vi "MecaDrivePoseEst2_Update.vi"(6 "Time":dbl=-1.0 format="%33.4f", 9 "module Positions":T1 {"RearRight" format="%19.3f"; "RearLeft" format="%19.3f"; "FrontRight" format="%19.3f"; "FrontLeft" format="%19.3f"}, 10 "GyroAngle":T4={"VALUE"=0.0, "COS"=1.0, "SIN"=0.0} {"SIN" format="%13.4f"; "COS" format="%13.4f"; "VALUE" format="%13.4f"}, 11 "in MecaDrivePoseEstimate":T5={"M_Vision_K"=[], "m_nominal_dT"=0.0, "m_PrevTime_Sec"=0.0, "Pose_Buffer"={"TimeStamps"=[], "DataArray"=[], "Min_TimeStamp"=0.0, "Max_TimeStamp"=0.0, "ItemCount"=0, "MaxBufferTime"=0.0}, "Meca_Drive_Odom"={"POSE"={"TRANSLATION"={"X"=0.0, "Y"=0.0}, "ROTATION"={"VALUE"=0.0, "COS"=1.0, "SIN"=0.0}}, "GyroOffset"={"VALUE"=0.0, "COS"=1.0, "SIN"=0.0}, "PreviousAngle"={"VALUE"=0.0, "COS"=1.0, "SIN"=0.0}, "Kinematics"={"FrontLeft"={"X"=0.0, "Y"=0.0}, "FrontRight"={"X"=0.0, "Y"=0.0}, "RearLeft"={"X"=0.0, "Y"=0.0}, "RearRight"={"X"=0.0, "Y"=0.0}, "InverseKinematics"=[[0.0, 1.0, -1.0, 0.0], [0.0, 1.0, 1.0, 0.0], [0.0, 1.0, 1.0, 0.0], [0.0, 1.0, -1.0, 0.0]], "ForwardKinematics"=[[0.0, 1.0, -1.0, 0.0], [0.0, 1.0, 1.0, 0.0], [0.0, 1.0, 1.0, 0.0], [0.0, 1.0, -1.0, 0.0]], "PrevCoR"={"X"=0.0, "Y"=0.0}}, "PreviousWheelPositions"={"FrontLeft"=0.0, "FrontRight"=0.0, "RearLeft"=0.0, "RearRight"=0.0, "P"=FALSE}}, "M_Q"=[[0.0], [0.0], [0.0]]} {"Meca_Drive_Odom"."PreviousWheelPositions"."RearRight" format="%19.3f"; "Meca_Drive_Odom"."PreviousWheelPositions"."RearLeft" format="%19.3f"; "Meca_Drive_Odom"."PreviousWheelPositions"."FrontRight" format="%19.3f"; "Meca_Drive_Odom"."PreviousWheelPositions"."FrontLeft" format="%19.3f"; "Meca_Drive_Odom"."Kinematics"."PrevCoR"."Y" format="%14.3f"; "Meca_Drive_Odom"."Kinematics"."PrevCoR"."X" format="%14.3f"; "Meca_Drive_Odom"."Kinematics"."RearRight"."Y" format="%14.3f"; "Meca_Drive_Odom"."Kinematics"."RearRight"."X" format="%14.3f"; "Meca_Drive_Odom"."Kinematics"."RearLeft"."Y" format="%14.3f"; "Meca_Drive_Odom"."Kinematics"."RearLeft"."X" format="%14.3f"; "Meca_Drive_Odom"."Kinematics"."FrontRight"."Y" format="%14.3f"; "Meca_Drive_Odom"."Kinematics"."FrontRight"."X" format="%14.3f"; "Meca_Drive_Odom"."Kinematics"."FrontLeft"."Y" format="%14.3f"; "Meca_Drive_Odom"."Kinematics"."FrontLeft"."X" format="%14.3f"; "Meca_Drive_Odom"."PreviousAngle"."SIN" format="%13.4f"; "Meca_Drive_Odom"."PreviousAngle"."COS" format="%13.4f"; "Meca_Drive_Odom"."PreviousAngle"."VALUE" format="%13.4f"; "Meca_Drive_Odom"."GyroOffset"."SIN" format="%13.4f"; "Meca_Drive_Odom"."GyroOffset"."COS" format="%13.4f"; "Meca_Drive_Odom"."GyroOffset"."VALUE" format="%13.4f"; "Meca_Drive_Odom"."POSE"."ROTATION"."SIN" format="%13.4f"; "Meca_Drive_Odom"."POSE"."ROTATION"."COS" format="%13.4f"; "Meca_Drive_Odom"."POSE"."ROTATION"."VALUE" format="%13.4f"; "Meca_Drive_Odom"."POSE"."TRANSLATION"."Y" format="%14.3f"; "Meca_Drive_Odom"."POSE"."TRANSLATION"."X" format="%14.3f"}) -> (0 "Error":bool, 2 "Estimated Pose":T2 {"ROTATION"."SIN" format="%13.4f"; "ROTATION"."COS" format="%13.4f"; "ROTATION"."VALUE" format="%13.4f"; "TRANSLATION"."Y" format="%14.3f"; "TRANSLATION"."X" format="%14.3f"}, 3 "Out MecaDrivePoseEstimate":T5={"M_Vision_K"=[], "m_nominal_dT"=0.0, "m_PrevTime_Sec"=0.0, "Pose_Buffer"={"TimeStamps"=[], "DataArray"=[], "Min_TimeStamp"=0.0, "Max_TimeStamp"=0.0, "ItemCount"=0, "MaxBufferTime"=0.0}, "Meca_Drive_Odom"={"POSE"={"TRANSLATION"={"X"=0.0, "Y"=0.0}, "ROTATION"={"VALUE"=0.0, "COS"=1.0, "SIN"=0.0}}, "GyroOffset"={"VALUE"=0.0, "COS"=1.0, "SIN"=0.0}, "PreviousAngle"={"VALUE"=0.0, "COS"=1.0, "SIN"=0.0}, "Kinematics"={"FrontLeft"={"X"=0.0, "Y"=0.0}, "FrontRight"={"X"=0.0, "Y"=0.0}, "RearLeft"={"X"=0.0, "Y"=0.0}, "RearRight"={"X"=0.0, "Y"=0.0}, "InverseKinematics"=[[0.0, 1.0, -1.0, 0.0], [0.0, 1.0, 1.0, 0.0], [0.0, 1.0, 1.0, 0.0], [0.0, 1.0, -1.0, 0.0]], "ForwardKinematics"=[[0.0, 1.0, -1.0, 0.0], [0.0, 1.0, 1.0, 0.0], [0.0, 1.0, 1.0, 0.0], [0.0, 1.0, -1.0, 0.0]], "PrevCoR"={"X"=0.0, "Y"=0.0}}, "PreviousWheelPositions"={"FrontLeft"=0.0, "FrontRight"=0.0, "RearLeft"=0.0, "RearRight"=0.0, "P"=FALSE}}, "M_Q"=[[0.0], [0.0], [0.0]]} {"Meca_Drive_Odom"."PreviousWheelPositions"."RearRight" format="%19.3f"; "Meca_Drive_Odom"."PreviousWheelPositions"."RearLeft" format="%19.3f"; "Meca_Drive_Odom"."PreviousWheelPositions"."FrontRight" format="%19.3f"; "Meca_Drive_Odom"."PreviousWheelPositions"."FrontLeft" format="%19.3f"; "Meca_Drive_Odom"."Kinematics"."PrevCoR"."Y" format="%14.3f"; "Meca_Drive_Odom"."Kinematics"."PrevCoR"."X" format="%14.3f"; "Meca_Drive_Odom"."Kinematics"."RearRight"."Y" format="%14.3f"; "Meca_Drive_Odom"."Kinematics"."RearRight"."X" format="%14.3f"; "Meca_Drive_Odom"."Kinematics"."RearLeft"."Y" format="%14.3f"; "Meca_Drive_Odom"."Kinematics"."RearLeft"."X" format="%14.3f"; "Meca_Drive_Odom"."Kinematics"."FrontRight"."Y" format="%14.3f"; "Meca_Drive_Odom"."Kinematics"."FrontRight"."X" format="%14.3f"; "Meca_Drive_Odom"."Kinematics"."FrontLeft"."Y" format="%14.3f"; "Meca_Drive_Odom"."Kinematics"."FrontLeft"."X" format="%14.3f"; "Meca_Drive_Odom"."PreviousAngle"."SIN" format="%13.4f"; "Meca_Drive_Odom"."PreviousAngle"."COS" format="%13.4f"; "Meca_Drive_Odom"."PreviousAngle"."VALUE" format="%13.4f"; "Meca_Drive_Odom"."GyroOffset"."SIN" format="%13.4f"; "Meca_Drive_Odom"."GyroOffset"."COS" format="%13.4f"; "Meca_Drive_Odom"."GyroOffset"."VALUE" format="%13.4f"; "Meca_Drive_Odom"."POSE"."ROTATION"."SIN" format="%13.4f"; "Meca_Drive_Odom"."POSE"."ROTATION"."COS" format="%13.4f"; "Meca_Drive_Odom"."POSE"."ROTATION"."VALUE" format="%13.4f"; "Meca_Drive_Odom"."POSE"."TRANSLATION"."Y" format="%14.3f"; "Meca_Drive_Odom"."POSE"."TRANSLATION"."X" format="%14.3f"})   [LabVIEW 2019, in "Trajectory_Library.lvlib"]
doc: "Updates the the robot odometry using only wheel encoder information. Note that this should be called every loop.\n\nInputs:\n - inSwerveDrivePoseEst -- system data cluster\n - gyroAngle -- The current gyro angle. (radians)\n - ModulePositions -- Array Module Position -- The current module positions (distance and angle)\n - currentTime -- Time at which this method was called, in seconds.\n\nOutputs:\n - outSwerveDrivePoseEst -- system data cluster\n - EstimatedPose -- The estimated pose of the robot in meters."
uses:
  Trajectory_Library.lvlib
  TypeDef/MECA_DRIVE_POSE_EST2.ctl
  <vilib>/Analysis/Matrix/Datatypes/RealMatrix.ctl
  TypeDef/TIME_INTERPOLATABLE_VARIANT.ctl
  TypeDef/MECA_DRIVE_ODOMETRY.ctl
  TypeDef/POSE2D.ctl
  TypeDef/TRANSLATION2D.ctl
  TypeDef/ROTATION2D.ctl
  TypeDef/MECA_DRIVE_KINEMATICS.ctl
  TypeDef/MECA_WHEEL_POSITIONS.ctl
  Util_GetTime_U32.vi
  Util_GetTime_U64.vi
  <vilib>/Analysis/Matrix/NI_Matrix.lvlib
panel:
  # "<3, 1>"
  # "<3, 3>"
  # "<3, 1>"
  # "<3, 3>"
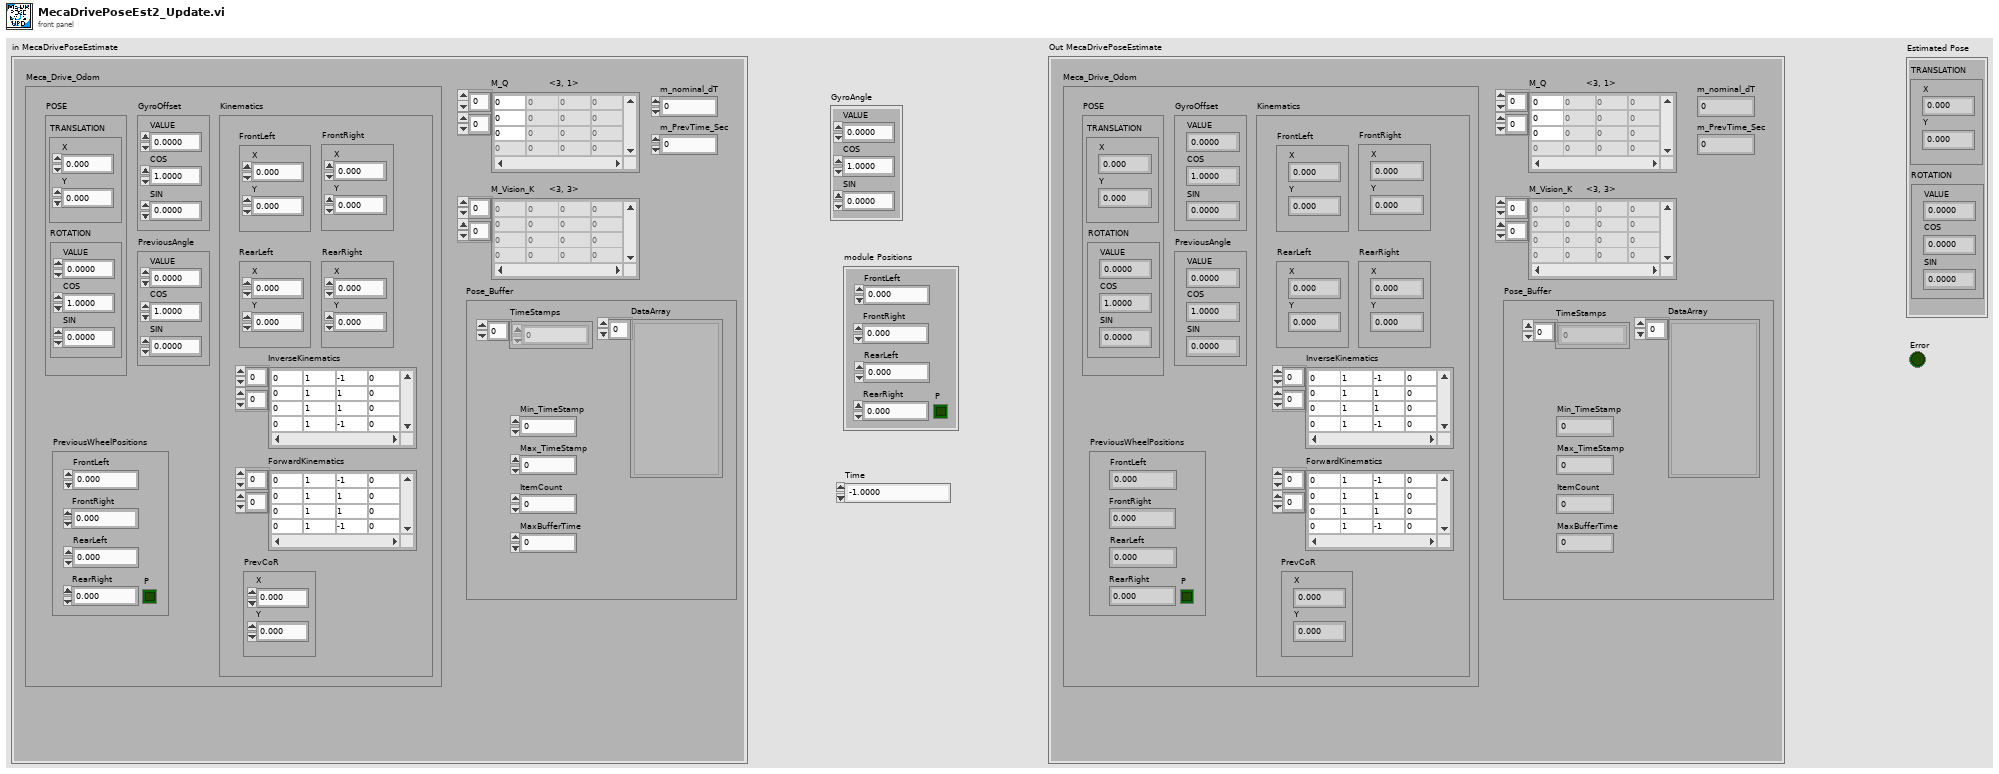
[diagram p1: front panel]
types:
  T1 = typedef "Trajectory_Library.lvlib/MECA_WHEEL_POSITIONS.ctl" = cluster{"FrontLeft":dbl, "FrontRight":dbl, "RearLeft":dbl, "RearRight":dbl, "P":bool}
  T2 = typedef "Trajectory_Library.lvlib/POSE2D.ctl" = cluster{"TRANSLATION":T3, "ROTATION":T4}
  T3 = typedef "Trajectory_Library.lvlib/TRANSLATION2D.ctl" = cluster{"X":dbl, "Y":dbl}
  T4 = typedef "Trajectory_Library.lvlib/ROTATION2D.ctl" = cluster{"VALUE":dbl, "COS":dbl, "SIN":dbl}
  T5 = typedef "Trajectory_Library.lvlib/MECA_DRIVE_POSE_EST2.ctl" = cluster{"M_Vision_K":T6, "m_nominal_dT":dbl, "m_PrevTime_Sec":dbl, "Pose_Buffer":T7, "Meca_Drive_Odom":T8, "M_Q":T6}
  T6 = typedef "NI_Matrix.lvlib/RealMatrix.ctl" = dbl[][]
  T7 = typedef "Trajectory_Library.lvlib/TIME_INTERPOLATABLE_VARIANT.ctl" = cluster{"TimeStamps":dbl[], "DataArray":variant[], "Min_TimeStamp":dbl, "Max_TimeStamp":dbl, "ItemCount":i32, "MaxBufferTime":dbl}
  T8 = typedef "Trajectory_Library.lvlib/MECA_DRIVE_ODOMETRY.ctl" = cluster{"POSE":T2, "GyroOffset":T4, "PreviousAngle":T4, "Kinematics":T9, "PreviousWheelPositions":T1}
  T9 = typedef "Trajectory_Library.lvlib/MECA_DRIVE_KINEMATICS.ctl" = cluster{"FrontLeft":T3, "FrontRight":T3, "RearLeft":T3, "RearRight":T3, "InverseKinematics":T6, "ForwardKinematics":T6, "PrevCoR":T3}
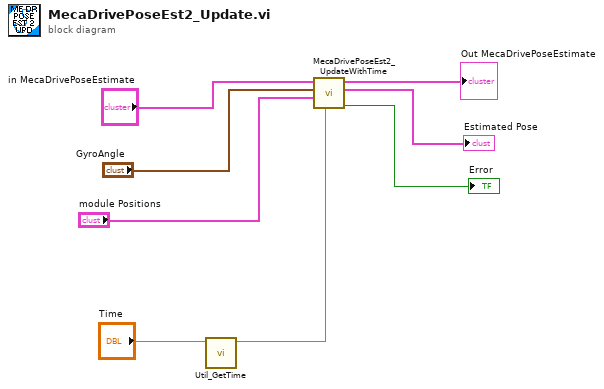
[diagram p0: block diagram]
diagram:
  n1 = call "Util_GetTime.vi"("Pass_Through_Time"="Time") -> ("FPGA_Time_Seconds"=w2:dbl)  [unwired: 8 in, 2 out]
  n2 = call "MecaDrivePoseEst2_UpdateWithTime.vi"("CurrentTimeSeconds"=w2, "module Positions"="module Positions", "GyroAngle"="GyroAngle", "in MecaDrivePoseEst2"="in MecaDrivePoseEstimate") -> ("Error"=→"Error":bool, "Estimated Pose"=→"Estimated Pose":T2, "Out MecaDrivePoseEst2"=→"Out MecaDrivePoseEstimate":T5)  [unwired: 5 in]
